vi "item select handle select commands.vi"(8 "error in (no error)":errorcluster, 10 "Action":T1, 11 "Loop data":T2) -> (0 "error out":errorcluster, 2 "New Selection states":bool[](array[boolean]), 3 "Loop data":T2)   [LabVIEW 2020, in "UI_ItemSelect.lvlib"]
uses:
  UI_ItemSelect.lvlib
  Tree item select loop data.ctl
  Item select ref type.ctl
  Tree item loop data.ctl
  Tree item selection indices.ctl
  checkbox state.ctl
  item select tree lock states.ctl
  item select action.ctl
  item select calc action.ctl
  <vilib>/Utility/error.llb/Error Cluster From Error Code.vi
  <vilib>/ErrorRing/Error Ring.xnode
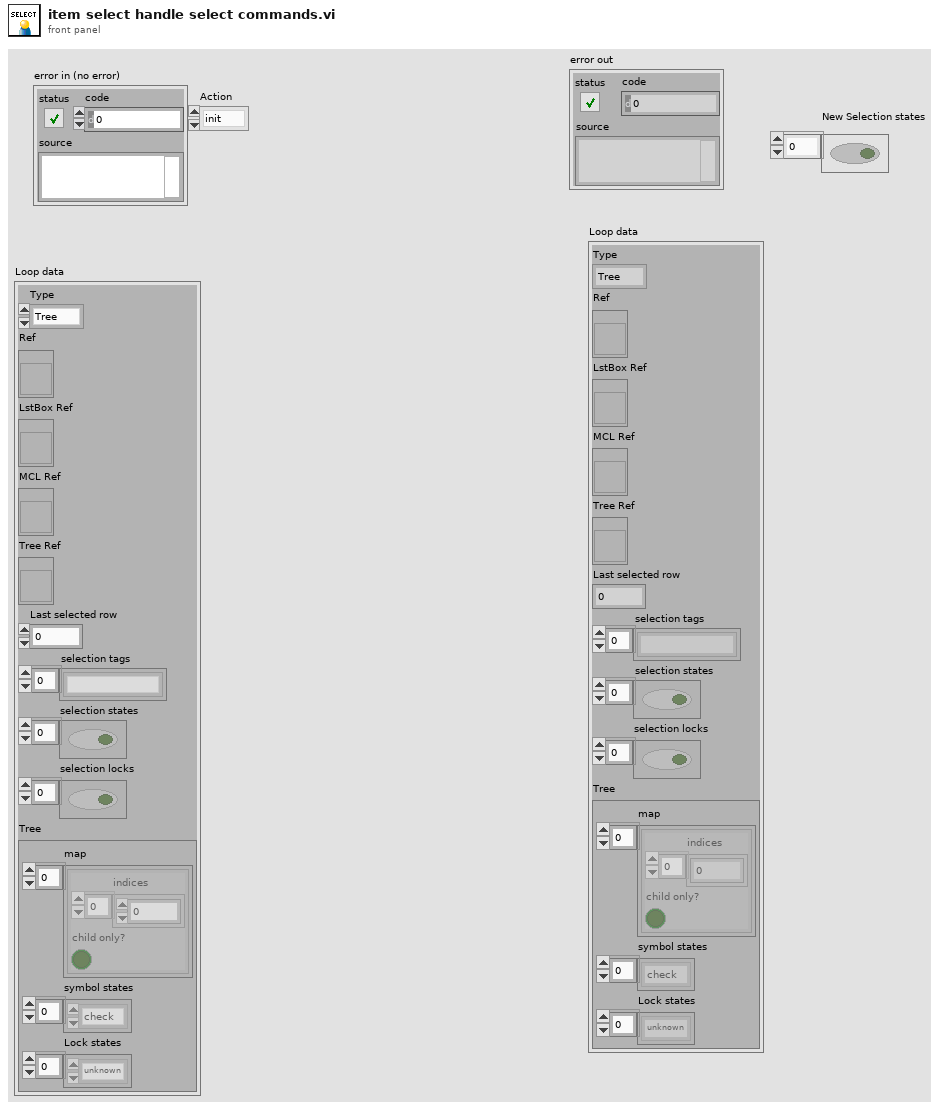
[diagram p1: front panel]
types:
  T1 = typedef "UI_ItemSelect.lvlib/item select action.ctl" = enum16{"init", "read", "write states", "write locks", "mouse down", "delete", "select all", "select none", "invert selection"}
  T2 = typedef "UI_ItemSelect.lvlib/Tree item select loop data.ctl" = cluster{"Type":T3, "Ref":refnum<vi>, "LstBox Ref":refnum<vi>, "MCL Ref":refnum<vi>, "Tree Ref":refnum<vi>, "Last selected row":i32, "selection tags":string[], "selection states":bool[], "selection locks":bool[], "Tree":T4}
  T3 = typedef "UI_ItemSelect.lvlib/Item select ref type.ctl" = enum16{"Tree", "MCL", "ListBox"}
  T4 = typedef "UI_ItemSelect.lvlib/Tree item loop data.ctl" = cluster{"map":T5[], "symbol states":T6[], "Lock states":T7[]}
  T5 = typedef "UI_ItemSelect.lvlib/Tree item selection indices.ctl" = cluster{"indices":i32[], "child only?":bool}
  T6 = typedef "UI_ItemSelect.lvlib/checkbox state.ctl" = enum16{"unknown", "check", "some", "no check"}
  T7 = typedef "UI_ItemSelect.lvlib/item select tree lock states.ctl" = enum16{"unknown", "locked", "unlocked"}
  T8 = typedef "UI_ItemSelect.lvlib/item select calc action.ctl" = enum16{"false", "true", "invert"}
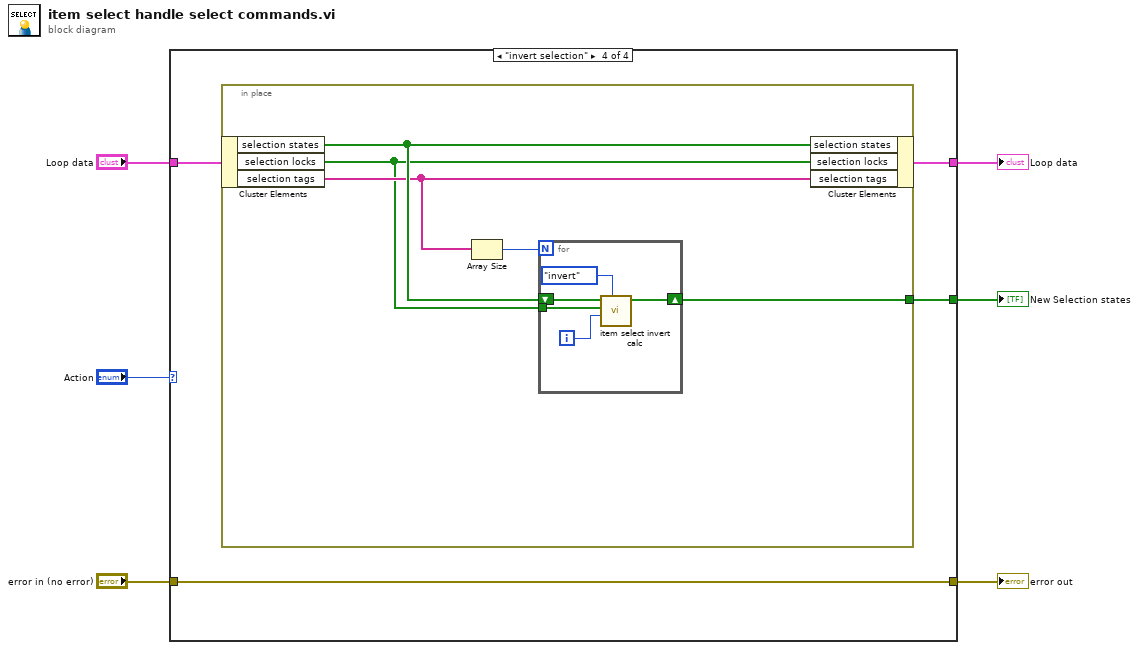
[diagram p0: block diagram]
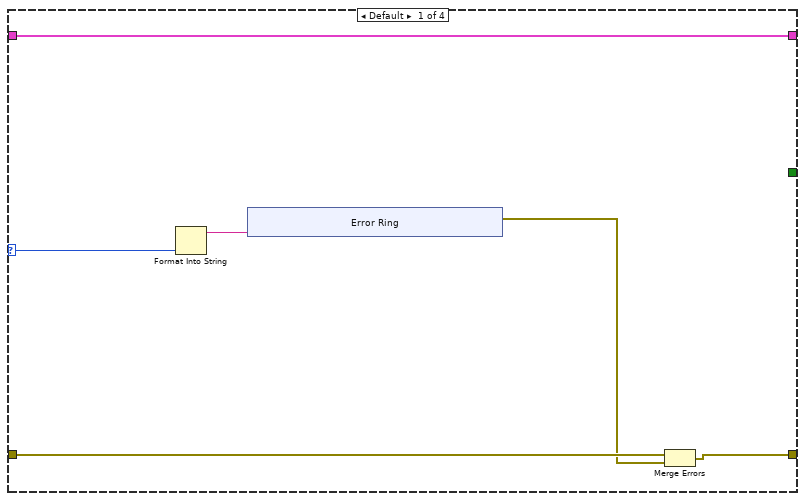
[diagram p2: hidden frame]
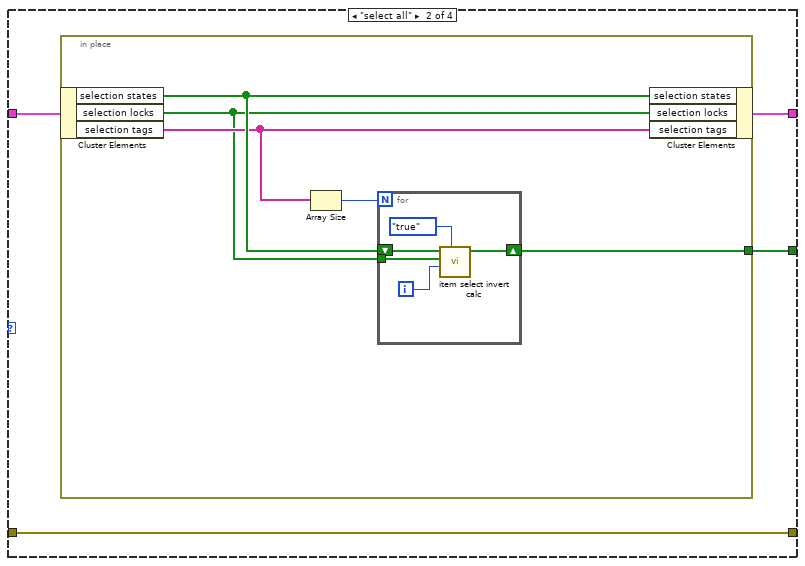
[diagram p3: hidden frame]
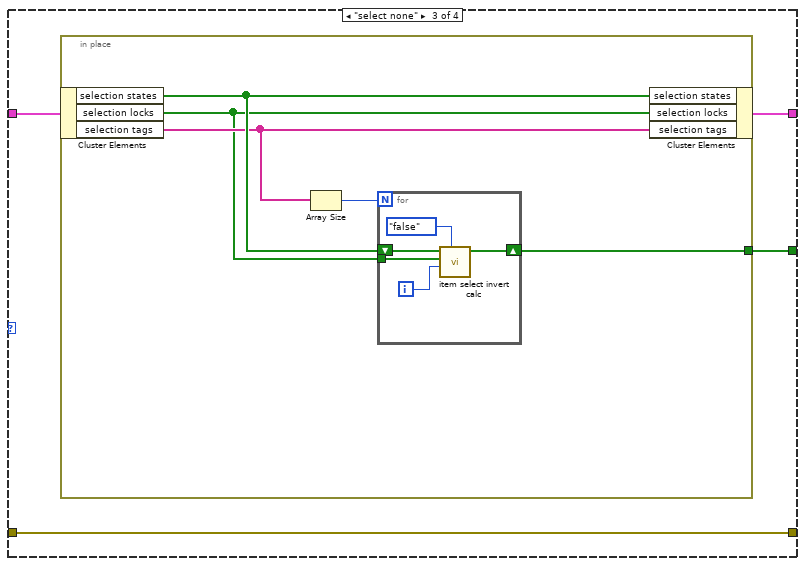
[diagram p4: hidden frame]
diagram:
  n1 = case shown="\"invert selection\"" "Action" {
    selector: "Action" -> [w12 _ _ _]
    tunnel: "Loop data" -> [w7 w23 w37 w51]
    tunnel: [_ w22 w36 w50] -> w4
    tunnel: [w7 w21 w35 w49] -> w3
    tunnel: "error in (no error)" -> [w10 w20 w34 w48]
    tunnel: [w8 w20 w34 w48] -> w1
    frame Default {
      n2 = Format Into String(w12) -> (resulting string=w11:string)  [unwired: 3 in, 1 out]
      n3 = xnode "Error Ring"("parameter 0"=w11) -> ("error out"=w9:errorcluster)
      n4 = Merge Errors(w10, w9) -> (w8:errorcluster)
    }
    frame "select all" {
      n5 = in-place {
        in-place-border: [w25] -> w22
        n6 = in-place-cluster #1(w23) -> ("selection states"=w28:bool[], "selection locks"=w26:bool[], "selection tags"=w27:string[])
        n7 = Array Size(array=w27) -> (size(s)=w24:i32)
        n8 = for {
          N: w24 -> [_]
          shift-right: [w31] -> w25
          shift-left: w28 -> [w33]
          tunnel: w26 -> [w32]
          i -> [w30]
          n9 = call "item select invert calc.vi"("Action"=item_select_calc_action."true", "selection index"=w30, "selection locks"=w32, "selection states"=w33) -> ("new selection states"=w31:bool[])  [unwired: 7 in]
        }
        n10 = in-place-cluster #1("selection states"=w28, "selection locks"=w26, "selection tags"=w27) -> (w21:T2)
      }
    }
    frame "select none" {
      n11 = in-place {
        in-place-border: [w39] -> w36
        n12 = in-place-cluster #2(w37) -> ("selection states"=w42:bool[], "selection locks"=w40:bool[], "selection tags"=w41:string[])
        n13 = Array Size(array=w41) -> (size(s)=w38:i32)
        n14 = for {
          N: w38 -> [_]
          shift-right: [w45] -> w39
          shift-left: w42 -> [w47]
          tunnel: w40 -> [w46]
          i -> [w44]
          n15 = call "item select invert calc.vi"("Action"=item_select_calc_action."false", "selection index"=w44, "selection locks"=w46, "selection states"=w47) -> ("new selection states"=w45:bool[])  [unwired: 7 in]
        }
        n16 = in-place-cluster #2("selection states"=w42, "selection locks"=w40, "selection tags"=w41) -> (w35:T2)
      }
    }
    frame "invert selection" {
      n17 = in-place {
        in-place-border: [w53] -> w50
        n18 = in-place-cluster #3(w51) -> ("selection states"=w56:bool[], "selection locks"=w54:bool[], "selection tags"=w55:string[])
        n19 = Array Size(array=w55) -> (size(s)=w52:i32)
        n20 = for {
          N: w52 -> [_]
          shift-right: [w59] -> w53
          shift-left: w56 -> [w61]
          tunnel: w54 -> [w60]
          i -> [w58]
          n21 = call "item select invert calc.vi"("Action"=item_select_calc_action."invert", "selection index"=w58, "selection locks"=w60, "selection states"=w61) -> ("new selection states"=w59:bool[])  [unwired: 7 in]
        }
        n22 = in-place-cluster #3("selection states"=w56, "selection locks"=w54, "selection tags"=w55) -> (w49:T2)
      }
    }
  }
  "Loop data" <- w3
  "error out" <- w1
  "New Selection states" <- w4
